vi "chart show blanks as.vi"(8 "error in (no error)":errorcluster, 10 "option":u8, 11 "chart":u32) -> (0 "error out":errorcluster)   [LabVIEW 8.6]
doc: "void chart_show_blanks_as(lxw_chart chart, uint8_t option);"
uses:
  pending_lvxlsxwriter/xlsxwriter.dll
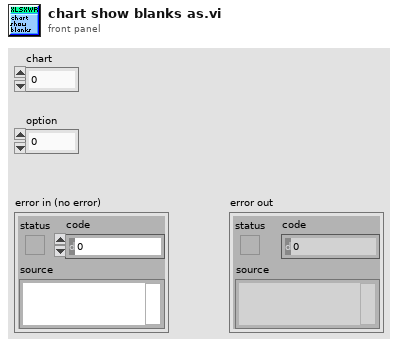
[diagram p1: front panel]
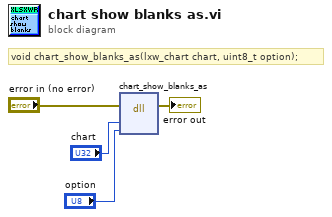
[diagram p0: block diagram]
diagram:
  # "void chart_show_blanks_as(lxw_chart chart, uint8_t option);"
  n1 = dll-call lib="C:/Users/WDAGUtilityAccount/Desktop/pending_lvxlsxwriter/xlsxwriter.*" fn="chart_show_blanks_as"(error in="error in (no error)", "chart"="chart", "option"="option") -> (error out=→"error out":errorcluster)  [unwired: 5 in, 1 out]
